vi "Open_URL.vi"(11 "URL":string) -> ()   [LabVIEW 2018]
panel:
  in  "WebBrowser":refnum<k7>(container) caption="网页浏览器"
types:
  T1 = enum32{"Invalid", "Standard", "Closed", "Hidden", "Minimized", "Maximized"}
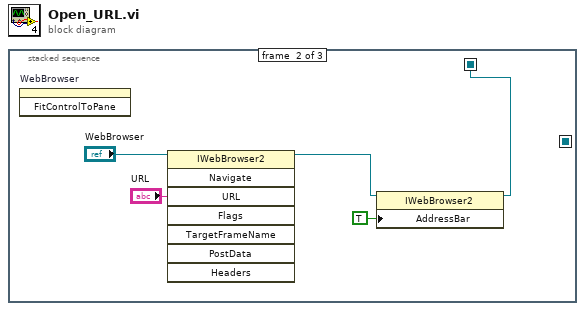
[diagram p0: block diagram]
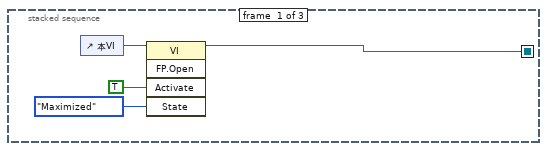
[diagram p2: hidden frame]
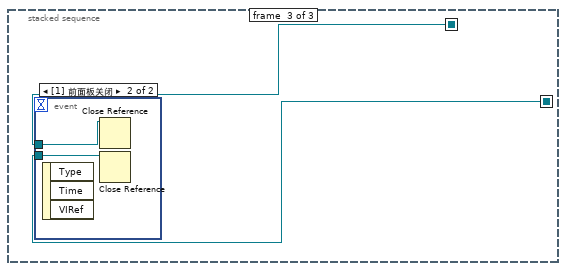
[diagram p3: hidden frame]
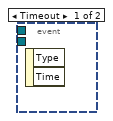
[diagram p4: hidden frame]
diagram:
  n1 = stacked-sequence {
    seq-local: [_ w5 _] -> [_ _ w11]
    seq-local: [w1 _ _] -> [_ _ w10]
    frame #0 {
      n2 = control-ref of="本VI"() -> (w4:refnum<vi>)
      n3 = invoke class="VI" method="FP.Open"(reference=w4, "Activate"=TRUE ("激活？"), "State"=T1."Maximized" ("状态")) -> (reference out=w1:refnum<vi>)  [unwired: 2 in, 4 out]
    }
    frame #1 {
      n4 = invoke on="WebBrowser" class="AXCont" method="FitControlToPane"() -> ()  [unwired: 3 in, 3 out]
      n5 = invoke class="IWebBrowser2" method="Navigate"(reference="WebBrowser", "URL"="URL") -> (reference out=w7:refnum<k7>)  [unwired: 6 in, 7 out]
      n6 = property class="IWebBrowser2"(reference=w7, "AddressBar"=TRUE) -> (reference out=w5:refnum<k7>)  [unwired: 1 in, 1 out]
    }
    frame #2 {
      n7 = event shown="[1] 前面板关闭" {
        selector: _ -> [_ _]
        dyn-events: _ -> [_ _]
        timeout: _ -> [_ _]
        tunnel: w11 -> [_ w13]
        tunnel: w10 -> [_ w12]
        event Timeout {
          n8 = event-data() -> ()  [unwired: 1 in, 2 out]
        }
        event Panel Close {
          n9 = event-data() -> ()  [unwired: 1 in, 3 out]
          n10 = Close Reference(reference=w13) -> ()  [unwired: 1 in, 1 out]
          n11 = Close Reference(reference=w12) -> ()  [unwired: 1 in, 1 out]
        }
      }
    }
  }
